vi "GetConnectedPads.vi"(8 "Error In":errorcluster, 9 "Pad Number":i32, 10 "Input Index":i32, 11 "Card In":cluster{"Session":u32, "Card number":u32}) -> (0 "Error Out":errorcluster, 2 "Pads":u32[](array[numeric]), 3 "Card Out":cluster{"Session":u32, "Card number":u32})   [LabVIEW 2012, in "Virtual-PGA.lvlib"]
uses:
  Virtual-PGA.lvlib
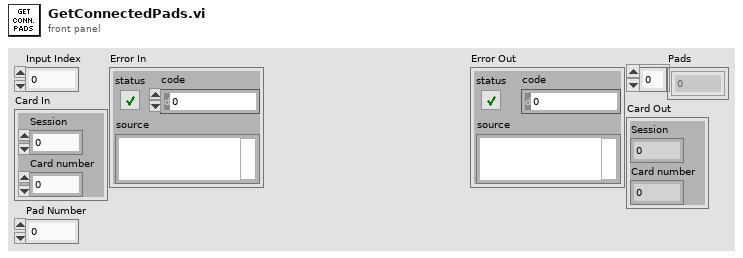
[diagram p1: front panel]
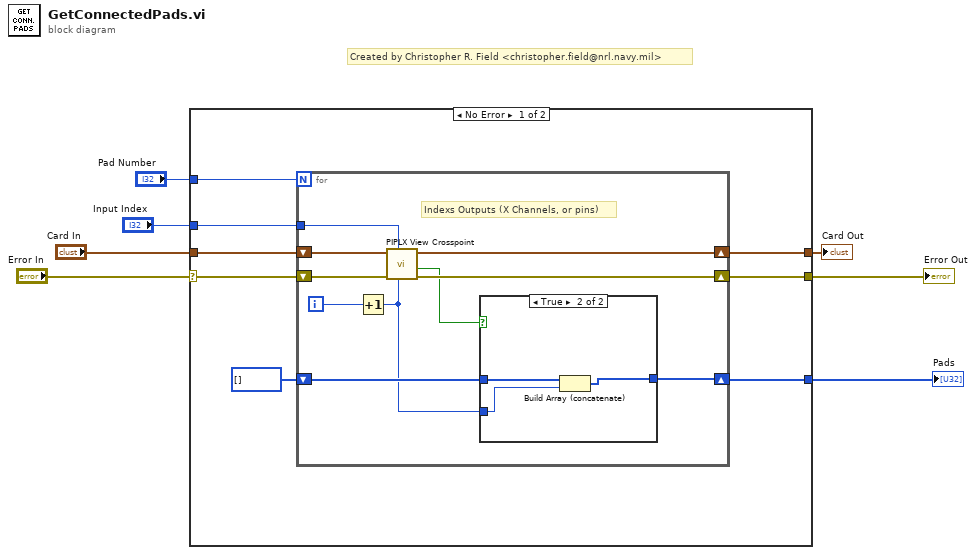
[diagram p0: block diagram]
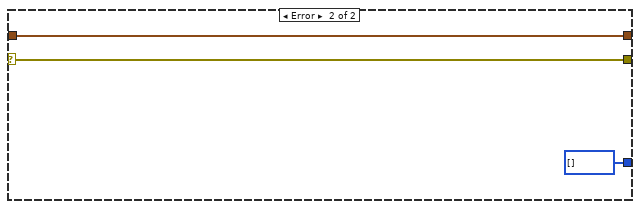
[diagram p3: hidden frame]
diagram:
  # "Created by Christopher R. Field <christopher.field@nrl.navy.mil>"
  n1 = case shown="No Error" "Error In" {
    selector: "Error In" -> [w9 w32]
    tunnel: "Input Index" -> [w14 _]
    tunnel: "Card In" -> [w13 w31]
    tunnel: [w12 u32[] []] -> w5
    tunnel: "Pad Number" -> [w11 _]
    tunnel: [w10 w32] -> w3
    tunnel: [w8 w31] -> w1
    frame No Error {
      n2 = for {
        N: w11 -> [_]
        tunnel: w14 -> [w22]
        shift-right: [w17] -> w12
        shift-left: u32[] [] -> [w19]
        shift-right: [w24] -> w10
        shift-left: w9 -> [w25]
        shift-right: [w16] -> w8
        shift-left: w13 -> [w23]
        i -> [w21]
        # "Indexs Outputs (X Channels, or pins)"
        n3 = Increment(x=w21) -> (x+1=w18:i32)
        n4 = call <instrlib>:"PIPLX View Crosspoint.vi"("Column"=w18, "Row"=w22, "error in"=w25, "Input Handle"=w23) -> ("error out"=w24:errorcluster, "State"=w20:bool, "Output Handle"=w16:cluster{"Session":u32, "Card number":u32})  [unwired: 5 in]
        n5 = case shown="True" w20 {
          tunnel: w19 -> [w26 w29]
          tunnel: w18 -> [_ w28]
          tunnel: [w26 w27] -> w17
          frame False {
          }
          frame True {
            n6 = Build Array (concatenate)(w29, w28) -> (w27:u32[])
          }
        }
      }
    }
    frame Error {
    }
  }
  "Error Out" <- w3
  "Pads" <- w5
  "Card Out" <- w1
